vi "target.vi"() -> ()   [LabVIEW 2020]
uses:
  <vilib>/Platform/TimedLoop/XDataNode/timing_clust.ctl
  <vilib>/Platform/TimedLoop/XDataNode/nitl_modes.ctl
  <vilib>/Platform/TimedLoop/XDataNode/wakeup.ctl
  <vilib>/Analysis/Matrix/Numeric/Conversions/Array To Matrix - RA.vi
  <vilib>/Analysis/Matrix/Numeric/Conversions/Array To Matrix - RA2.vi
  <vilib>/Analysis/Matrix/Numeric/Conversions/Matrix To Array - RM.vi
  <vilib>/platform/TimedLoop/XDataNode/XDataNode.xnode
  <vilib>/Platform/TimedLoop/XDataNode/XDNodeRunTimeDep.lvlib
  <vilib>/Analysis/Matrix/NI_Matrix.lvlib
panel:
  out "Error":errorcluster
  in  "ms per read sample":dbl
  out "Analog in":dbl
  out "Waveform Chart":dbl(graph)
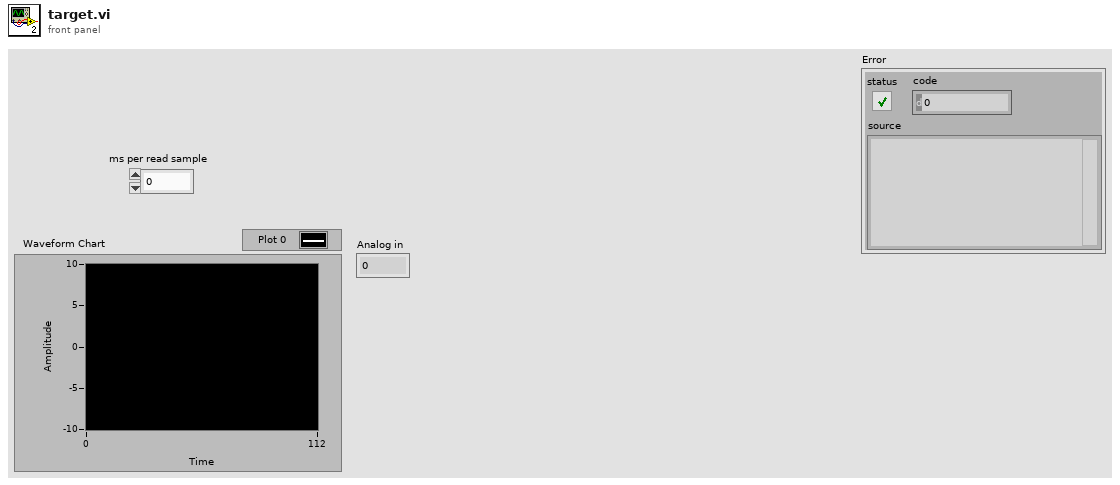
[diagram p1: front panel]
types:
  T1 = typedef "NI_Matrix.lvlib/RealMatrix.ctl" = dbl[][]
  T2 = typedef "XDNodeRunTimeDep.lvlib/timing_clust.ctl" = cluster{"Expected End [f-1]":u64, "Actual End [f-1]":u64, "Finished Late? [f-1]":bool, "Expected End [i-1]":u64, "Actual End [i-1]":u64, "Finished Late? [i-1]":bool, "Expected Start [i]":u64, "Actual Start [i]":u64, "Expected Start [f]":u64, "Actual Start [f]":u64, "Source Name":string, "Structure Name":string, "Period":i64, "Deadline":i64, "Offset":i64, "Start":i64, "Priority":i32, "Timeout":i32, "Mode":T3, "Wakeup Reason":T4, "Error":errorcluster, "Source Type":string, "Secondary Source Type":string, "Global End Time":u64, "Global Start Time":u64, "Frame Duration":u64, "Iteration Duration":u64, "Assigned CPU":i32, "I/O Scan Engine Mode":u32}
  T3 = typedef "XDNodeRunTimeDep.lvlib/nitl_modes.ctl" = enum32{"No Change", "Process missed periods, maintain original phase", "Discard missed periods, maintain original phase", "Process missed periods, ignore original phase", "Discard missed periods, ignore original phase"}
  T4 = typedef "XDNodeRunTimeDep.lvlib/wakeup.ctl" = enum32{"Normal", "Aborted", "Asynchronous wakeup", "Timing source error", "Timed loop error", "Timeout"}
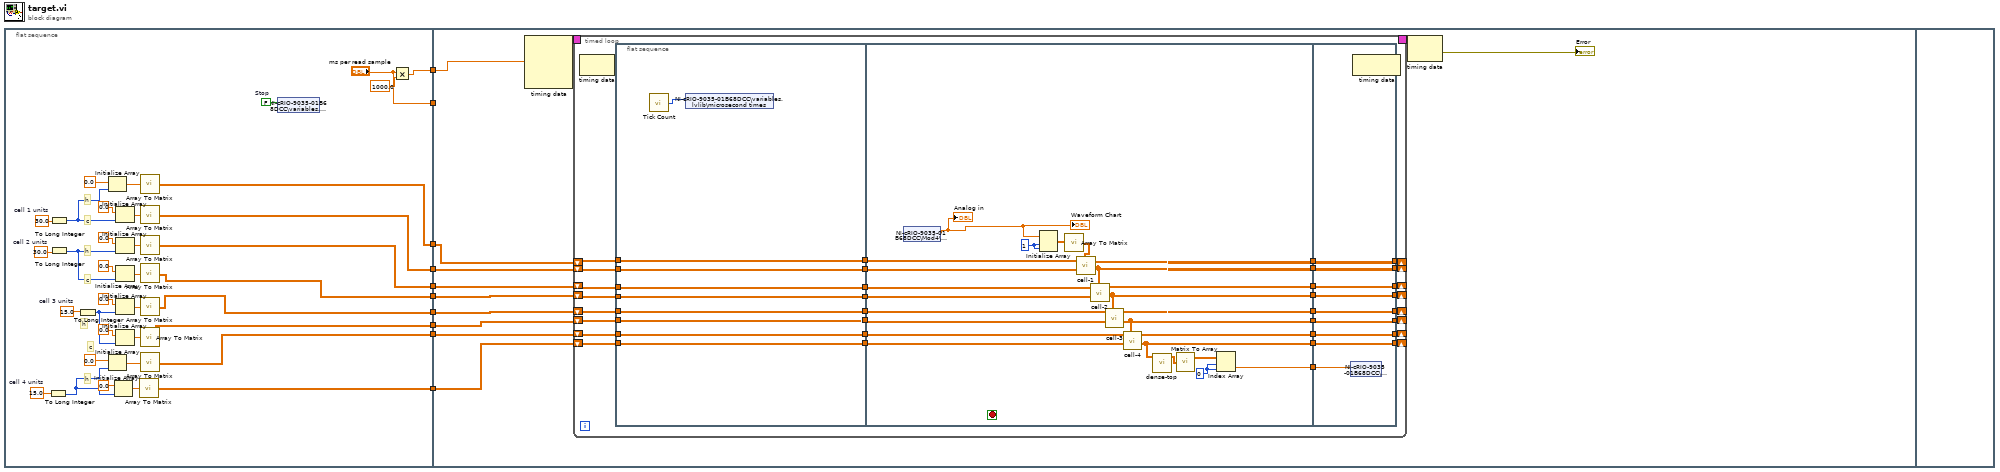
[diagram p0: block diagram]
diagram:
  n1 = flat-sequence {
    tunnel: [w44] -> w10
    tunnel: [w20] -> w9
    tunnel: [w19] -> w8
    tunnel: [w18] -> w7
    tunnel: [w17] -> w6
    tunnel: [w16] -> w5
    tunnel: [w15] -> w4
    tunnel: [w14] -> w3
    tunnel: [w13] -> w2
    tunnel: ["ms per read sample"] -> w1
    tunnel: w10 -> [w56]
    tunnel: w9 -> [w55]
    tunnel: w8 -> [w54]
    tunnel: w7 -> [w53]
    tunnel: w6 -> [w52]
    tunnel: w5 -> [w51]
    tunnel: w4 -> [w50]
    tunnel: w3 -> [w49]
    tunnel: w2 -> [w48]
    tunnel: w1 -> [_]
    frame #0 {
      w28 = 15.0  # cell 4 units
      w26 = 15.0  # cell 3 units
      w24 = 30.0  # cell 2 units
      w22 = 30.0  # cell 1 units
      w46 = FALSE  # Stop
      # "c"
      # "c"
      # "c"
      # "h"
      # "h"
      # "h"
      # "h"
      n2 = To Long Integer(number=w28) -> (32bit integer=w11:i32)
      n3 = To Long Integer(number=w22) -> (32bit integer=w38:i32)
      n4 = To Long Integer(number=w24) -> (32bit integer=w40:i32)
      n5 = To Long Integer(number=w26) -> (32bit integer=w42:i32)
      n6 = Initialize Array(0.0, w38) -> (w37:dbl[])
      n7 = Initialize Array(0.0, w11) -> (w43:dbl[])
      n8 = Initialize Array(0.0, w11) -> (w36:dbl[])
      n9 = Initialize Array(0.0, w38) -> (w33:dbl[])
      n10 = Initialize Array(0.0, w40) -> (w39:dbl[])
      n11 = Initialize Array(0.0, w40) -> (w34:dbl[])
      n12 = Initialize Array(0.0, w42) -> (w41:dbl[])
      n13 = Initialize Array(0.0, w42) -> (w35:dbl[])
      n14 = call-poly <vilib>:"Array To Matrix.vi"("Real 1D Array"=w36) -> ("Real Matrix (Column Vector)"=w13:T1)
      n15 = call-poly <vilib>:"Array To Matrix.vi"("Real 1D Array"=w37) -> ("Real Matrix (Column Vector)"=w20:T1)
      n16 = call-poly <vilib>:"Array To Matrix.vi"("Real 1D Array"=w33) -> ("Real Matrix (Column Vector)"=w19:T1)
      n17 = call-poly <vilib>:"Array To Matrix.vi"("Real 1D Array"=w39) -> ("Real Matrix (Column Vector)"=w18:T1)
      n18 = call-poly <vilib>:"Array To Matrix.vi"("Real 1D Array"=w34) -> ("Real Matrix (Column Vector)"=w17:T1)
      n19 = call-poly <vilib>:"Array To Matrix.vi"("Real 1D Array"=w41) -> ("Real Matrix (Column Vector)"=w16:T1)
      n20 = call-poly <vilib>:"Array To Matrix.vi"("Real 1D Array"=w35) -> ("Real Matrix (Column Vector)"=w15:T1)
      n21 = call-poly <vilib>:"Array To Matrix.vi"("Real 1D Array"=w43) -> ("Real Matrix (Column Vector)"=w14:T1)
      n22 = shared-variable "NI-cRIO-9035-01B68DCC\\variables.lvlib\\Stop"(w46) -> ()  [unwired: 1 in, 1 out]
      n23 = Multiply(x="ms per read sample", y=1000.0) -> (x*y=w44:dbl)
    }
    frame #1 {
      n24 = node-c288(w56) -> (w58:T2)  [unwired: 3 in]
      n25 = timed-loop {
        timing: w58 -> [_]
        timing-out: [_] -> w57
        shift-right: [w91] -> _
        shift-left: w55 -> [w90]
        shift-right: [w89] -> _
        shift-left: w54 -> [w88]
        shift-right: [w87] -> _
        shift-left: w53 -> [w86]
        shift-right: [w85] -> _
        shift-left: w52 -> [w84]
        shift-right: [w83] -> _
        shift-left: w51 -> [w82]
        shift-right: [w81] -> _
        shift-left: w50 -> [w80]
        shift-right: [w79] -> _
        shift-left: w49 -> [w78]
        shift-right: [w77] -> _
        shift-left: w48 -> [w76]
        stop <- _ stop-if-true
        n26 = node-c288() -> ()  [unwired: 1 in, 1 out]
        n27 = flat-sequence {
          tunnel: w76 -> [w93]
          tunnel: w78 -> [w94]
          tunnel: w80 -> [w95]
          tunnel: w82 -> [w96]
          tunnel: w84 -> [w97]
          tunnel: w86 -> [w98]
          tunnel: w88 -> [w99]
          tunnel: w90 -> [w100]
          tunnel: [w100] -> w75
          tunnel: [w99] -> w74
          tunnel: [w98] -> w73
          tunnel: [w97] -> w72
          tunnel: [w96] -> w71
          tunnel: [w95] -> w70
          tunnel: [w94] -> w69
          tunnel: [w93] -> w68
          tunnel: w75 -> [w116]
          tunnel: w74 -> [w114]
          tunnel: w73 -> [w112]
          tunnel: w72 -> [w110]
          tunnel: w71 -> [w108]
          tunnel: w70 -> [w106]
          tunnel: w69 -> [w104]
          tunnel: w68 -> [w102]
          tunnel: [w117] -> w67
          tunnel: [w115] -> w66
          tunnel: [w113] -> w65
          tunnel: [w111] -> w64
          tunnel: [w109] -> w63
          tunnel: [w107] -> w62
          tunnel: [w105] -> w61
          tunnel: [w103] -> w60
          tunnel: [w101] -> w59
          tunnel: [w126] -> w77
          tunnel: [w127] -> w79
          tunnel: [w128] -> w81
          tunnel: [w129] -> w83
          tunnel: [w130] -> w85
          tunnel: [w131] -> w87
          tunnel: [w132] -> w89
          tunnel: [w133] -> w91
          tunnel: w67 -> [w133]
          tunnel: w66 -> [w132]
          tunnel: w65 -> [w131]
          tunnel: w64 -> [w130]
          tunnel: w63 -> [w129]
          tunnel: w62 -> [w128]
          tunnel: w61 -> [w127]
          tunnel: w60 -> [w126]
          tunnel: w59 -> [w125]
          frame #0 {
            n28 = call "Tick Count"() -> ("Tick Count(uSec)"=w92:u32)
            n29 = shared-variable "NI-cRIO-9035-01B68DCC\\variables.lvlib\\microsecond times"(w92) -> ()  [unwired: 1 in, 1 out]
          }
          frame #1 {
            w123 = 0
            w119 = 1
            n30 = shared-variable "NI-cRIO-9035-01B68DCC\\Mod4\\AI0"() -> (w118:dbl)  [unwired: 1 in, 1 out]
            "Analog in" <- w118
            "Waveform Chart" <- w118
            n31 = Initialize Array(w118, w119, w119) -> (w120:dbl[][])
            n32 = call-poly <vilib>:"Array To Matrix.vi"("Real 2D Array"=w120) -> ("Real Matrix"=w121:T1)
            n33 = call "cell-1.vi"("x"=w121, "h"=w114, "c"=w116) -> ("h + 1"=w115:T1, "c + 1"=w117:T1)  [unwired: 7 in]
            n34 = call "cell-2.vi"("x"=w115, "h"=w110, "c"=w112) -> ("h + 1"=w111:T1, "c + 1"=w113:T1)  [unwired: 7 in]
            n35 = call "cell-3.vi"("x"=w111, "h"=w106, "c"=w108) -> ("h + 1"=w107:T1, "c + 1"=w109:T1)  [unwired: 7 in]
            n36 = call "cell-4.vi"("x"=w107, "h"=w102, "c"=w104) -> ("h + 1"=w103:T1, "c + 1"=w105:T1)  [unwired: 7 in]
            n37 = call "dense-top.vi"("x_dense"=w103) -> ("y_out"=w124:T1)  [unwired: 10 in]
            n38 = call-poly <vilib>:"Matrix To Array.vi"("Real Matrix"=w124) -> ("Real 2D Array"=w122:dbl[][])
            n39 = Index Array(array=w122, index (row)=w123, index (col)=w123) -> (element=w101:dbl)
          }
          frame #2 {
            n40 = shared-variable "NI-cRIO-9035-01B68DCC\\variables.lvlib\\y"(w125) -> ()  [unwired: 1 in, 1 out]
          }
        }
        n41 = node-c288() -> ()  [unwired: 1 in, 1 out]
      }
      n42 = node-c288(w57) -> (→"Error":errorcluster)
    }
    frame #2 {
    }
  }
